vi "final_control_mk11_060325.vi"() -> ()   [LabVIEW 2023]
doc: "Simplified example program for initializing the COM port, determining the data frame of up to 26 Alicats, acquiring the data of the same number of Alicats, displaying the data of the one with the selected unit ID, and writing a setpoint to the same selected unit ID.\n\nThis is a slightly more feature rich version of the Alicat Simplified Driver Example, and contains an example of a method for interfacing with up to 26 Alicats on a single COM port by means of for loops with shift registers to handle sequential commands to each included Alicat. This also contains a method to write a setpoint to the same selected unit.\n\nIf coding for multiple Alicats on a single COM port without the use of for loops with shift registers, ensure that each Alicat command is executed sequentially. Alicat's RS-232/485 does not work if multiple devices are responding simultaneously."
uses:
  <vilib>/Platform/TimedLoop/XDataNode/timing_clust.ctl
  <vilib>/Platform/TimedLoop/XDataNode/nitl_modes.ctl
  <vilib>/Platform/TimedLoop/XDataNode/wakeup.ctl
  <vilib>/DAQmx/write.llb/DAQmx Write (Analog 1D DBL NChan 1Samp).vi
  <vilib>/DAQmx/read.llb/DAQmx Read (Analog DBL 1Chan 1Samp).vi
  <extravilib>/ChannelInstances/Tag-bool/Read With Abort.vi
  <extravilib>/ChannelInstances/Tag-bool/Write With Abort.vi
  <vilib>/Utility/file.llb/Write Delimited Spreadsheet (string).vi
  <extravilib>/ChannelInstances/Tag-bool/Instantiate.vi
  <vilib>/Utility/file.llb/Read Delimited Spreadsheet (DBL).vi
  <extravilib>/ChannelInstances/Tag-bool/EndpointRead.vi
  <vilib>/DAQmx/miscellaneous.llb/DAQmx Fill In Error Info.vi
  <extravilib>/ChannelInstances/Tag-bool/Endpoint.vi
  <vilib>/platform/TimedLoop/XDataNode/XDataNode.xnode
  <vilib>/express/express arith-compare/Formula/XNode/ExpressFormulaBlockNode.xnode
  <vilib>/Platform/TimedLoop/XDataNode/XDNodeRunTimeDep.lvlib
  <extravilib>/ChannelInstances/Tag-bool.lvlib
panel:
  in  "Tab Control":enum32{"Page 1", "Page 2"}(tab)
  in  "COM Port Settings":T1={"Baud Rate"=enum."19200", "VISA Sesssion In"="MassFlowControllers"}
  out "Range Exceeded":bool
  out "Error Present":bool
  out "Error Text":string
  out "Elapsed Time [ms]\n(all units)":dbl caption="Elapsed Time (s)"
  in  "Minimum time between \nreadings [ms] (all units)":u32
  in  "Device ID's \nto Include:":T2={"A"=TRUE, "B"=TRUE, "C"=TRUE, "D"=TRUE, "E"=TRUE, "F"=TRUE, "G"=FALSE, "H"=FALSE, "I"=FALSE, "J"=FALSE, "K"=FALSE, "L"=FALSE, "M"=FALSE, "N"=FALSE, "O"=FALSE, "P"=FALSE, "Q"=FALSE, "R"=FALSE, "S"=FALSE, "T"=FALSE, "U"=FALSE, "V"=FALSE, "W"=FALSE, "X"=FALSE, "Y"=FALSE, "Z"=FALSE}
  out "Active Device":u16(ring) items=["A", "B", "C", "D", "E", "F"]
  out "Meas. Data (for active device)":T3
  in  "Write File":path
  in  "Hold Time\n[min]":dbl=17.0 min=17.0
  out "N":i32
  in  "Read File":path
  in  "End Program":bool
  in  "Start From:":i32=1
  in  "t_read [ms]":dbl=24000.0
  out "T_SCh [C]":dbl format="%0.2f"
  out "iter start":string
  out "Iter_Duration [ms]":string
  out "C_SP [ppm]":string
  out "C_H2 [ppm]":string
  in  "Start Times":path
  in  "API Key":string="V1WFARF28XTM5DW7"
  out "len_SP":i32
  out "Setpoints":dbl[][](array[numeric])=[[4.2, 3.3], [69.0, 4.2]]
  out "Z":dbl[](array[numeric])
  out "ASP":dbl
  out "BSP":dbl
  out "CSP":dbl
  out "DSP":dbl
  out "ESP":dbl
  out "FSP":dbl
  out "N_read":i32
  out "Iter_#":string
  out "V_D":string
  out "V_H":string
  out "all rows":dbl[][](array[numeric])
  out "T_SCh":string
  out "Iteration Duration":i64
  out "read_cnt_true":i32
  out "iter_dur_read [ms]":i64
  out "t_diff":dbl
  out "date":string
  out "time":string
  # "Totalizer Timer"
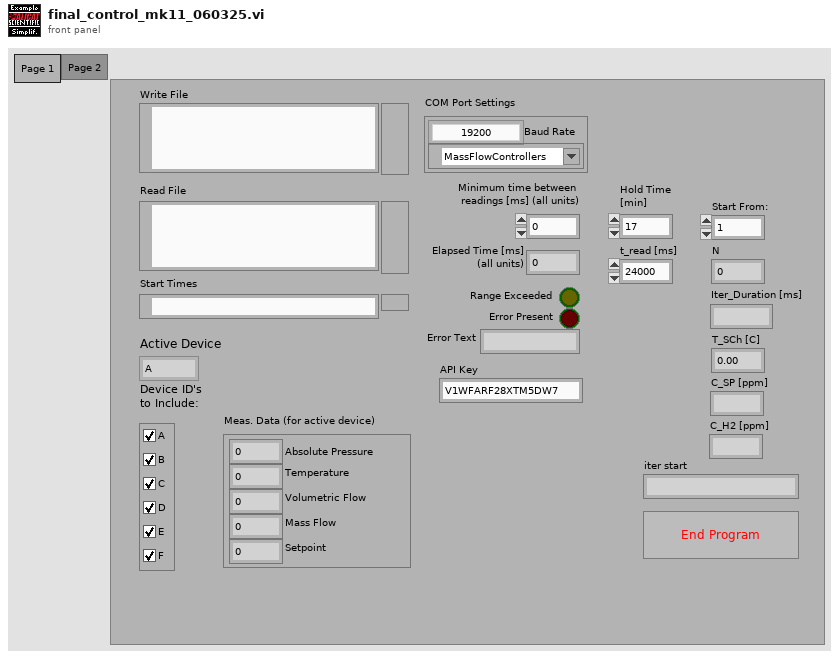
[diagram p1: front panel]
types:
  T1 = cluster{"Baud Rate":enum8{"2400", "9600", "19200", "38400", "57600", "115200", "Unknown"}, "VISA Sesssion In":refnum<visa-resource-name>}
  T2 = cluster{"A":bool, "B":bool, "C":bool, "D":bool, "E":bool, "F":bool, "G":bool, "H":bool, "I":bool, "J":bool, "K":bool, "L":bool, "M":bool, "N":bool, "O":bool, "P":bool, "Q":bool, "R":bool, "S":bool, "T":bool, "U":bool, "V":bool, "W":bool, "X":bool, "Y":bool, "Z":bool}
  T3 = cluster{"Absolute Pressure":dbl, "Gauge/Diff. Pressure":dbl, "Barometric Pressure":dbl, "Temperature":dbl, "Volumetric Flow":dbl, "Mass Flow":dbl, "Setpoint":dbl, "Valve Drive":dbl, "Totalizer":dbl, "[hr]":dbl, "[min]":dbl, "[sec]":dbl, "Totalizer Average Flow":dbl, "Totalizer Peak Flow":dbl, "Gas selected":string}
  T4 = cluster{"Unit ID":string, "Baud Rate":enum8{"2400", "9600", "19200", "38400", "57600", "115200", "Unknown"}, "VISA Sesssion In":refnum<visa-resource-name>}
  T5 = enum16{"Request Ack", "Set Setpoint", "Set Lo Limit", "Set Hi Limit", "Set Prop Band 0-99.9", "Set Integral 0-9.99", "Set Derivative 0-5.0", "Read Int Temp", "Read Ext Temp", "Read Setpoint", "Read Low Limit", "Read High Limit", "Read Prop Band", "Read Integral", "Read Derivative "}
  T6 = typedef "XDNodeRunTimeDep.lvlib/timing_clust.ctl" = cluster{"Expected End [f-1]":u64, "Actual End [f-1]":u64, "Finished Late? [f-1]":bool, "Expected End [i-1]":u64, "Actual End [i-1]":u64, "Finished Late? [i-1]":bool, "Expected Start [i]":u64, "Actual Start [i]":u64, "Expected Start [f]":u64, "Actual Start [f]":u64, "Source Name":string, "Structure Name":string, "Period":i64, "Deadline":i64, "Offset":i64, "Start":i64, "Priority":i32, "Timeout":i32, "Mode":T7, "Wakeup Reason":T8, "Error":errorcluster, "Source Type":string, "Secondary Source Type":string, "Global End Time":u64, "Global Start Time":u64, "Frame Duration":u64, "Iteration Duration":u64, "Assigned CPU":i32, "I/O Scan Engine Mode":u32}
  T7 = typedef "XDNodeRunTimeDep.lvlib/nitl_modes.ctl" = enum32{"No Change", "Process missed periods, maintain original phase", "Discard missed periods, maintain original phase", "Process missed periods, ignore original phase", "Discard missed periods, ignore original phase"}
  T8 = typedef "XDNodeRunTimeDep.lvlib/wakeup.ctl" = enum32{"Normal", "Aborted", "Asynchronous wakeup", "Timing source error", "Timed loop error", "Timeout"}
  T9 = typedef "Tag-bool.lvlib/))Channel.ctl" = refnum<queue>
  T10 = enum8{"2400", "9600", "19200", "38400", "57600", "115200", "Unknown"}
  T11 = cluster{"Absolute Pressure":bool, "Gauge/Diff. Pressure":bool, "Barometric Pressure":bool, "Temperature":bool, "Volumetric":bool, "Mass":bool, "Setpoint":bool, "Valve Drive":bool, "Totalizer":bool, "Totalizer Timer":bool, "Totalizer Average Flow":bool, "Totalizer Peak Flow":bool, "Gas Selected":bool, "Tot. Timer Format":u16}
  T12 = cluster{"Controller Full Scale":dbl, "Controller Select":u16, "Control Range":enum16{"Normal", "Inverted", "Bidirectional", "Unknown"}}
  T13 = cluster{"Controller Full Scale":dbl, "Controller Select":u16, "Control Range":enum16{"Normal", "Inverted", "Bidirectional", "Unknown"}}[]
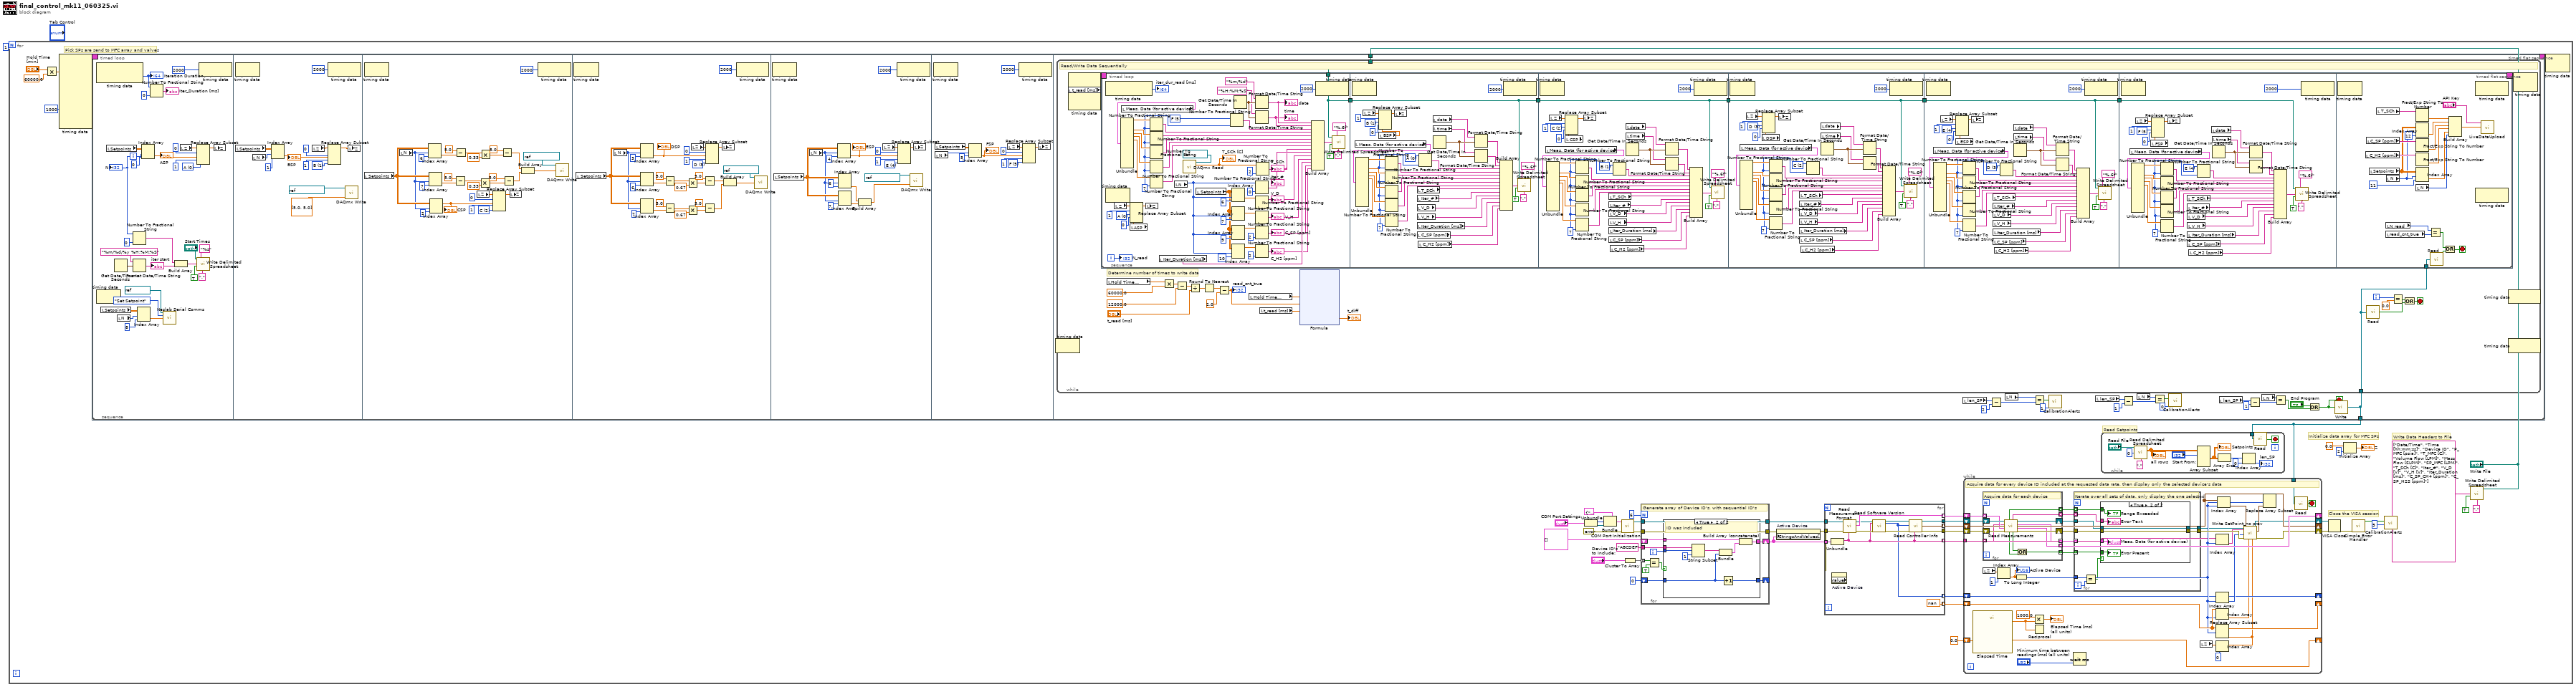
[diagram p0: block diagram]
diagram:
  n1 = for {
    N: 1 -> [_]
    # "Pick SPs are send to MFC array and valves"
    # "Write Data Headers to File"
    # "Read Setpoints"
    # "Initialize data array for MFC SPs"
    # "Close the VISA session"
    n2 = Multiply(x="Hold Time\n[min]", y=60000.0) -> (x*y=w5:dbl)
    n3 = node-c288(w5, i64 1000 ("Offset")) -> (w46:T6)  [unwired: 8 in]
    n4 = timed-loop "Write Data" {
      timing: w46 -> [_]
      timing-out: [_] -> w45
      tunnel: [w59] -> w12
      tunnel: "Write File" -> [w58]
      i -> [w73]
      stop <- w227 stop-if-true
      n5 = timed-sequence {
        timing: _ -> [_]
        timing-out: _ -> [_]
        tunnel: [w61] -> w59
        tunnel: w58 -> [w60]
        n6 = timed-flat-sequence {
          tunnel: [w222] -> w61
          tunnel: w60 -> [w223]
          frame #0 {
            w83 = u16 0 items=["A", "B", "C", "D", "E", "F"]
            n7 = node-c288() -> (w77:i64)  [unwired: 1 in, 1 out]
            "Iteration Duration" <- w77
            n8 = local read "Setpoints"() -> (w67:dbl[][])
            n9 = local read "Setpoints"() -> (w90:dbl[][])
            n10 = Get Date/Time In Seconds() -> (seconds since 1Jan1904=w78:timestamp)
            n11 = local read "N"() -> (w66:i32)
            n12 = Number To Fractional String(number=w73, precision (6)=i16 0) -> (F-format string=w71:string)  [unwired: 2 in]
            n13 = Format Date/Time String(time format string (%c)="%m/%d/%y %H:%M:%S", seconds (now)=w78) -> (date/time string=w70:string)  [unwired: 1 in]
            "iter start" <- w70
            n14 = Index Array(array=w67, index (row)=w66, index (col)=8 ("disabled index (col)")) -> (element=w64:dbl)
            n15 = Index Array(array=w90, index (row)=w73, index (col)=0 ("index (row)")) -> (element=w88:dbl)
            "ASP" <- w88
            n16 = Number To Fractional String(number=w77, precision (6)=i16 0) -> (F-format string=→"Iter_Duration [ms]":string)  [unwired: 2 in]
            n17 = call "Neslab Serial Comms.vi"("VISA resource name"=refnum<visa-resource-name> "COM1", "Command"=T5."Set Setpoint", "Set Value"=w64) -> ()  [unwired: 6 in, 7 out]
            n18 = Build Array(w71, w70) -> (w69:string[])
            n19 = local read "Z"() -> (w86:dbl[])
            n20 = Replace Array Subset(array=w86, new element #1=w88, index #1=0 ("index"), new element #2=w83, index #2=1 ("index")) -> (w87:dbl[])
            n21 = call-poly <vilib>:"Write Delimited Spreadsheet.vi"("file path (dialog if empty)"="Start Times", "format (%s)"="%s" ("format (%.3f)"), "1D data"=w69, "append to file? (new file:F)"=TRUE, "delimiter (\\t)"="," ("delimiter (\\t)")) -> ()  [unwired: 9 in, 2 out]
            n22 = node-c288(i64 2000 ("Start")) -> ()  [unwired: 1 out]
            n23 = local write "Z"(w87) -> ()
            "N" <- w73
          }
          frame #1 {
            w98 = u16 1 items=["A", "B", "C", "D", "E", "F"]
            n24 = node-c288() -> ()  [unwired: 1 in, 1 out]
            n25 = local read "Setpoints"() -> (w106:dbl[][])
            n26 = local read "N"() -> (w99:i32)
            n27 = Index Array(array=w106, index (row)=w99, index (col)=1 ("index (row)")) -> (element=w103:dbl)
            "BSP" <- w103
            n28 = local read "Z"() -> (w101:dbl[])
            n29 = Replace Array Subset(array=w101, new element #1=w103, index #1=0 ("index"), new element #2=w98, index #2=1 ("index")) -> (w102:dbl[])
            n30 = node-c288(i64 2000 ("Start")) -> ()  [unwired: 1 out]
            n31 = call-poly <vilib>:"DAQmx Write.vi"("task/channels in"=refnum<k21> "Valve_cont", "data"=dbl[] [5.0, 5.0]) -> ()  [unwired: 11 in, 3 out]
            n32 = local write "Z"(w102) -> ()
          }
          frame #2 {
            w113 = u16 2 items=["A", "B", "C", "D", "E", "F"]
            n33 = node-c288() -> ()  [unwired: 1 in, 1 out]
            n34 = local read "Setpoints"() -> (w125:dbl[][])
            n35 = local read "N"() -> (w124:i32)
            n36 = Index Array(array=w125, index (row)=w124, index (col)=6 ("disabled index (col)")) -> (element=w115:dbl)
            n37 = Index Array(array=w125, index (row)=w124, index (col)=7 ("disabled index (col)")) -> (element=w123:dbl)
            n38 = Index Array(array=w125, index (row)=w124, index (col)=2 ("index (row)")) -> (element=w137:dbl)
            "CSP" <- w137
            n39 = Subtract(x=5.0, y=w123) -> (x-y=w132:dbl)
            n40 = Subtract(x=5.0, y=w115) -> (x-y=w119:dbl)
            n41 = local read "Z"() -> (w135:dbl[])
            n42 = Multiply(x=w132, y=0.33) -> (x*y=w130:dbl)
            n43 = Multiply(x=w119, y=0.33) -> (x*y=w117:dbl)
            n44 = Replace Array Subset(array=w135, new element #1=w137, index #1=0 ("index"), new element #2=w113, index #2=1 ("index")) -> (w136:dbl[])
            n45 = Subtract(x=5.0, y=w117) -> (x-y=w114:dbl)
            n46 = Subtract(x=5.0, y=w130) -> (x-y=w127:dbl)
            n47 = local write "Z"(w136) -> ()
            n48 = Build Array(w114, w127) -> (w126:dbl[])
            n49 = node-c288(i64 2000 ("Start")) -> ()  [unwired: 1 out]
            n50 = call-poly <vilib>:"DAQmx Write.vi"("task/channels in"=refnum<k21> "Valve_cont", "data"=w126) -> ()  [unwired: 11 in, 3 out]
          }
          frame #3 {
            w164 = u16 3 items=["A", "B", "C", "D", "E", "F"]
            n51 = node-c288() -> ()  [unwired: 1 in, 1 out]
            n52 = local read "Setpoints"() -> (w153:dbl[][])
            n53 = local read "N"() -> (w152:i32)
            n54 = Index Array(array=w153, index (row)=w152, index (col)=7 ("disabled index (col)")) -> (element=w145:dbl)
            n55 = Index Array(array=w153, index (row)=w152, index (col)=3 ("index (row)")) -> (element=w168:dbl)
            "DSP" <- w168
            n56 = Index Array(array=w153, index (row)=w152, index (col)=6 ("disabled index (col)")) -> (element=w151:dbl)
            n57 = Subtract(x=5.0, y=w151) -> (x-y=w161:dbl)
            n58 = Subtract(x=5.0, y=w145) -> (x-y=w149:dbl)
            n59 = Multiply(x=w161, y=0.67) -> (x*y=w159:dbl)
            n60 = Multiply(x=w149, y=0.67) -> (x*y=w147:dbl)
            n61 = local read "Z"() -> (w166:dbl[])
            n62 = Subtract(x=5.0, y=w159) -> (x-y=w155:dbl)
            n63 = Subtract(x=5.0, y=w147) -> (x-y=w144:dbl)
            n64 = Replace Array Subset(array=w166, new element #1=w168, index #1=0 ("index"), new element #2=w164, index #2=1 ("index")) -> (w167:dbl[])
            n65 = local write "Z"(w167) -> ()
            n66 = Build Array(w155, w144) -> (w154:dbl[])
            n67 = node-c288(i64 2000 ("Start")) -> ()  [unwired: 1 out]
            n68 = call-poly <vilib>:"DAQmx Write.vi"("task/channels in"=refnum<k21> "Valve_cont", "data"=w154) -> ()  [unwired: 11 in, 3 out]
          }
          frame #4 {
            w185 = u16 4 items=["A", "B", "C", "D", "E", "F"]
            n69 = node-c288() -> ()  [unwired: 1 in, 1 out]
            n70 = local read "Setpoints"() -> (w180:dbl[][])
            n71 = local read "N"() -> (w179:i32)
            n72 = Index Array(array=w180, index (row)=w179, index (col)=4 ("index (row)")) -> (element=w189:dbl)
            "ESP" <- w189
            n73 = Index Array(array=w180, index (row)=w179, index (col)=6 ("disabled index (col)")) -> (element=w182:dbl)
            n74 = Index Array(array=w180, index (row)=w179, index (col)=7 ("disabled index (col)")) -> (element=w181:dbl)
            n75 = Build Array(w182, w181) -> (w178:dbl[])
            n76 = local read "Z"() -> (w187:dbl[])
            n77 = node-c288(i64 2000 ("Start")) -> ()  [unwired: 1 out]
            n78 = Replace Array Subset(array=w187, new element #1=w189, index #1=0 ("index"), new element #2=w185, index #2=1 ("index")) -> (w188:dbl[])
            n79 = call-poly <vilib>:"DAQmx Write.vi"("task/channels in"=refnum<k21> "Valve_cont", "data"=w178) -> ()  [unwired: 11 in, 3 out]
            n80 = local write "Z"(w188) -> ()
          }
          frame #5 {
            w199 = u16 5 items=["A", "B", "C", "D", "E", "F"]
            n81 = node-c288() -> ()  [unwired: 1 in, 1 out]
            n82 = local read "Setpoints"() -> (w202:dbl[][])
            n83 = local read "N"() -> (w197:i32)
            n84 = Index Array(array=w202, index (row)=w197, index (col)=5 ("index (row)")) -> (element=w198:dbl)
            "FSP" <- w198
            n85 = local read "Z"() -> (w201:dbl[])
            n86 = node-c288(i64 2000 ("Start")) -> ()  [unwired: 1 out]
            n87 = Replace Array Subset(array=w201, new element #1=w198, index #1=0 ("index"), new element #2=w199, index #2=1 ("index")) -> (w200:dbl[])
            n88 = local write "Z"(w200) -> ()
          }
          frame #6 {
            n89 = node-c288() -> ()  [unwired: 1 in, 1 out]
            n90 = local read "len_SP"() -> (w213:i32)
            n91 = Subtract(x=w213, y=2) -> (x-y=w215:i32)
            n92 = local read "N"() -> (w214:i32)
            n93 = Equal?(x=w214, y=w215) -> (x = y?=w211:bool)
            n94 = call "CalibrationAlerts.vi"("Alert Type (0)"=1, "Trigger"=w211) -> ()  [unwired: 10 in]
            n95 = local read "len_SP"() -> (w218:i32)
            n96 = Subtract(x=w218, y=1) -> (x-y=w217:i32)
            n97 = local read "N"() -> (w221:i32)
            n98 = Equal?(x=w221, y=w217) -> (x = y?=w210:bool)
            n99 = call "CalibrationAlerts.vi"("Alert Type (0)"=0, "Trigger"=w210) -> ()  [unwired: 10 in]
            n100 = local read "len_SP"() -> (w226:i32)
            n101 = Subtract(x=w226, y=1) -> (x-y=w229:i32)
            n102 = local read "N"() -> (w225:i32)
            n103 = Equal?(x=w225, y=w229) -> (x = y?=w228:bool)
            n104 = Or(x="End Program", y=w228) -> (x .or. y?=w227:bool)
            n105 = call <extravilib>:"Write.vi"("element"=w227) -> ("channel"=w222:T9)  [unwired: 1 out]
            n106 = while {
              tunnel: w223 -> [w251]
              tunnel: w222 -> [w241]
              i -> [w240]
              stop <- w247 stop-if-true
              # "Determine number of times to write data"
              # "Read/Write Data Sequentially"
              n107 = local read "t_read [ms]"() -> (w231:dbl)
              n108 = node-c288(w231) -> (w253:T6)  [unwired: 3 in]
              n109 = timed-loop {
                timing: w253 -> [_]
                timing-out: [_] -> w252
                tunnel: w251 -> [w266]
                tunnel: w241 -> [w267]
                i -> [w330]
                stop <- w564 stop-if-true
                n110 = timed-sequence {
                  timing: _ -> [_]
                  timing-out: _ -> [_]
                  tunnel: w267 -> [w269]
                  tunnel: w266 -> [w268]
                  n111 = timed-flat-sequence {
                    tunnel: [w296] -> w274
                    tunnel: w268 -> [w296]
                    tunnel: w274 -> [w361]
                    tunnel: [w361] -> w273
                    tunnel: w273 -> [w396]
                    tunnel: [w396] -> w272
                    tunnel: w272 -> [w434]
                    tunnel: [w434] -> w271
                    tunnel: w271 -> [w466]
                    tunnel: [w466] -> w270
                    tunnel: w270 -> [w519]
                    tunnel: w269 -> [w563]
                    frame #0 {
                      w311 = u16 5 items=["A", "B", "C", "D", "E", "F"]
                      w314 = u16 0 items=["A", "B", "C", "D", "E", "F"]
                      w307 = i16 7 ("precision (6)")
                      n112 = node-c288() -> (→"iter_dur_read [ms]":i64)  [unwired: 1 in]
                      n113 = local read "Z"() -> (w300:dbl[])
                      n114 = local read "Meas. Data (for active device)"() -> (w297:T3)
                      n115 = Unbundle(w297) -> ("Absolute Pressure"=w320:dbl, "Temperature"=w310:dbl, "Volumetric Flow"=w316:dbl, "Mass Flow"=w309:dbl, "Setpoint"=w308:dbl)  [unwired: 10 out]
                      n116 = local read "ASP"() -> (w298:dbl)
                      n117 = Replace Array Subset(array=w300, new element #1=w314, index #1=1 ("index"), new element #2=w298, index #2=0 ("index")) -> (w299:dbl[])
                      n118 = local write "Z"(w299) -> ()
                      n119 = Number To Fractional String(number=w320, precision (6)=w307) -> (F-format string=w305:string)  [unwired: 2 in]
                      n120 = Number To Fractional String(number=w310, precision (6)=w307) -> (F-format string=w303:string)  [unwired: 2 in]
                      n121 = Number To Fractional String(number=w316, precision (6)=w307) -> (F-format string=w304:string)  [unwired: 2 in]
                      n122 = Number To Fractional String(number=w309, precision (6)=w307) -> (F-format string=w302:string)  [unwired: 2 in]
                      n123 = Number To Fractional String(number=w308, precision (6)=w307) -> (F-format string=w301:string)  [unwired: 2 in]
                      n124 = local read "Iter_Duration [ms]"() -> (w295:string)
                      n125 = local read "N"() -> (w277:i32)
                      n126 = call-poly <vilib>:"DAQmx Read.vi"("task/channels in"=refnum<k21> "Temp") -> ("data"=w323:dbl)  [unwired: 12 in, 2 out]
                      "T_SCh [C]" <- w323
                      n127 = local read "Setpoints"() -> (w276:dbl[][])
                      n128 = Number To Fractional String(number=w311, precision (6)=w307) -> (F-format string=w306:string)  [unwired: 2 in]
                      n129 = Index Array(array=w276, index (row)=w277, index (col)=6 ("disabled index (col)")) -> (element=w327:dbl)
                      n130 = Index Array(array=w276, index (row)=w277, index (col)=7 ("disabled index (col)")) -> (element=w326:dbl)
                      n131 = Index Array(array=w276, index (row)=w277, index (col)=9 ("disabled index (col)")) -> (element=w283:dbl)
                      n132 = Index Array(array=w276, index (row)=w277, index (col)=10 ("disabled index (col)")) -> (element=w279:dbl)
                      n133 = Get Date/Time In Seconds() -> (seconds since 1Jan1904=w289:timestamp)
                      n134 = Format Date/Time String(time format string (%c)="%m/%d", seconds (now)=w289) -> (date/time string=w291:string)  [unwired: 1 in]
                      "date" <- w291
                      n135 = Format Date/Time String(time format string (%c)="%H:%M:%S", seconds (now)=w289) -> (date/time string=w290:string)  [unwired: 1 in]
                      "time" <- w290
                      n136 = Number To Fractional String(number=w277, precision (6)=i16 0) -> (F-format string=w292:string)  [unwired: 2 in]
                      "Iter_#" <- w292
                      n137 = Number To Fractional String(number=w327) -> (F-format string=w293:string)  [unwired: 3 in]
                      "V_D" <- w293
                      n138 = Number To Fractional String(number=w326) -> (F-format string=w294:string)  [unwired: 3 in]
                      "V_H" <- w294
                      n139 = Number To Fractional String(number=w283, precision (6)=i16 2) -> (F-format string=w281:string)  [unwired: 2 in]
                      "C_SP [ppm]" <- w281
                      n140 = Number To Fractional String(number=w279, precision (6)=i16 2) -> (F-format string=w275:string)  [unwired: 2 in]
                      "C_H2 [ppm]" <- w275
                      n141 = Number To Fractional String(number=w323, precision (6)=i16 2) -> (F-format string=w286:string)  [unwired: 2 in]
                      "T_SCh" <- w286
                      n142 = Build Array(w291, w290, w306, w305, w303, w304, w302, w301, w286, w292, w293, w294, w295, w281, w275) -> (w317:string[])
                      n143 = node-c288(i64 2000 ("Start")) -> ()  [unwired: 1 out]
                      n144 = call-poly <vilib>:"Write Delimited Spreadsheet.vi"("file path (dialog if empty)"=w296, "format (%s)"="%.6f" ("format (%.3f)"), "1D data"=w317, "append to file? (new file:F)"=TRUE, "delimiter (\\t)"="," ("delimiter (\\t)")) -> ()  [unwired: 9 in, 2 out]
                      "N_read" <- w330
                    }
                    frame #1 {
                      w358 = u16 0 items=["A", "B", "C", "D", "E", "F"]
                      w367 = u16 1 items=["A", "B", "C", "D", "E", "F"]
                      w354 = i16 7 ("precision (6)")
                      n145 = node-c288() -> ()  [unwired: 1 in, 1 out]
                      n146 = local read "Meas. Data (for active device)"() -> (w365:T3)
                      n147 = Unbundle(w365) -> ("Absolute Pressure"=w373:dbl, "Temperature"=w357:dbl, "Volumetric Flow"=w369:dbl, "Mass Flow"=w356:dbl, "Setpoint"=w355:dbl)  [unwired: 10 out]
                      n148 = local read "Z"() -> (w364:dbl[])
                      n149 = local read "BSP"() -> (w359:dbl)
                      n150 = Replace Array Subset(array=w364, new element #1=w367, index #1=1 ("index"), new element #2=w359, index #2=0 ("index")) -> (w363:dbl[])
                      n151 = Number To Fractional String(number=w373, precision (6)=w354) -> (F-format string=w352:string)  [unwired: 2 in]
                      n152 = Number To Fractional String(number=w357, precision (6)=w354) -> (F-format string=w350:string)  [unwired: 2 in]
                      n153 = Number To Fractional String(number=w369, precision (6)=w354) -> (F-format string=w351:string)  [unwired: 2 in]
                      n154 = Number To Fractional String(number=w356, precision (6)=w354) -> (F-format string=w349:string)  [unwired: 2 in]
                      n155 = Number To Fractional String(number=w355, precision (6)=w354) -> (F-format string=w348:string)  [unwired: 2 in]
                      n156 = local write "Z"(w363) -> ()
                      n157 = local read "T_SCh"() -> (w347:string)
                      n158 = local read "Iter_#"() -> (w346:string)
                      n159 = local read "V_D"() -> (w345:string)
                      n160 = local read "V_H"() -> (w344:string)
                      n161 = local read "Iter_Duration [ms]"() -> (w343:string)
                      n162 = local read "C_SP [ppm]"() -> (w337:string)
                      n163 = local read "C_H2 [ppm]"() -> (w336:string)
                      n164 = Number To Fractional String(number=w358, precision (6)=w354) -> (F-format string=w353:string)  [unwired: 2 in]
                      n165 = local read "date"() -> (w338:string)
                      n166 = local read "time"() -> (w339:string)
                      n167 = Get Date/Time In Seconds() -> (seconds since 1Jan1904=w340:timestamp)
                      n168 = Format Date/Time String(time format string (%c)=w338, seconds (now)=w340) -> (date/time string=w342:string)  [unwired: 1 in]
                      n169 = Format Date/Time String(time format string (%c)=w339, seconds (now)=w340) -> (date/time string=w341:string)  [unwired: 1 in]
                      n170 = Build Array(w342, w341, w353, w352, w350, w351, w349, w348, w347, w346, w345, w344, w343, w337, w336) -> (w370:string[])
                      n171 = node-c288(i64 2000 ("Start")) -> ()  [unwired: 1 out]
                      n172 = call-poly <vilib>:"Write Delimited Spreadsheet.vi"("file path (dialog if empty)"=w361, "format (%s)"="%.6f" ("format (%.3f)"), "1D data"=w370, "append to file? (new file:F)"=TRUE, "delimiter (\\t)"="," ("delimiter (\\t)")) -> ()  [unwired: 9 in, 2 out]
                    }
                    frame #2 {
                      w402 = u16 1 items=["A", "B", "C", "D", "E", "F"]
                      w401 = i16 7 ("precision (6)")
                      w414 = u16 2 items=["A", "B", "C", "D", "E", "F"]
                      n173 = node-c288() -> ()  [unwired: 1 in, 1 out]
                      n174 = local read "Meas. Data (for active device)"() -> (w403:T3)
                      n175 = Unbundle(w403) -> ("Absolute Pressure"=w408:dbl, "Temperature"=w406:dbl, "Volumetric Flow"=w407:dbl, "Mass Flow"=w405:dbl, "Setpoint"=w404:dbl)  [unwired: 10 out]
                      n176 = local read "Z"() -> (w413:dbl[])
                      n177 = local read "CSP"() -> (w409:dbl)
                      n178 = Replace Array Subset(array=w413, new element #1=w414, index #1=1 ("index"), new element #2=w409, index #2=0 ("index")) -> (w412:dbl[])
                      n179 = Number To Fractional String(number=w408, precision (6)=w401) -> (F-format string=w389:string)  [unwired: 2 in]
                      n180 = Number To Fractional String(number=w406, precision (6)=w401) -> (F-format string=w388:string)  [unwired: 2 in]
                      n181 = Number To Fractional String(number=w407, precision (6)=w401) -> (F-format string=w387:string)  [unwired: 2 in]
                      n182 = Number To Fractional String(number=w405, precision (6)=w401) -> (F-format string=w386:string)  [unwired: 2 in]
                      n183 = Number To Fractional String(number=w404, precision (6)=w401) -> (F-format string=w385:string)  [unwired: 2 in]
                      n184 = local write "Z"(w412) -> ()
                      n185 = local read "T_SCh"() -> (w395:string)
                      n186 = local read "Iter_#"() -> (w394:string)
                      n187 = local read "V_D"() -> (w393:string)
                      n188 = local read "V_H"() -> (w392:string)
                      n189 = local read "Iter_Duration [ms]"() -> (w391:string)
                      n190 = local read "C_SP [ppm]"() -> (w379:string)
                      n191 = local read "C_H2 [ppm]"() -> (w378:string)
                      n192 = Number To Fractional String(number=w402, precision (6)=w401) -> (F-format string=w390:string)  [unwired: 2 in]
                      n193 = local read "date"() -> (w380:string)
                      n194 = local read "time"() -> (w381:string)
                      n195 = Get Date/Time In Seconds() -> (seconds since 1Jan1904=w382:timestamp)
                      n196 = Format Date/Time String(time format string (%c)=w380, seconds (now)=w382) -> (date/time string=w384:string)  [unwired: 1 in]
                      n197 = Format Date/Time String(time format string (%c)=w381, seconds (now)=w382) -> (date/time string=w383:string)  [unwired: 1 in]
                      n198 = Build Array(w384, w383, w390, w389, w388, w387, w386, w385, w395, w394, w393, w392, w391, w379, w378) -> (w397:string[])
                      n199 = node-c288(i64 2000 ("Start")) -> ()  [unwired: 1 out]
                      n200 = call-poly <vilib>:"Write Delimited Spreadsheet.vi"("file path (dialog if empty)"=w396, "format (%s)"="%.6f" ("format (%.3f)"), "1D data"=w397, "append to file? (new file:F)"=TRUE, "delimiter (\\t)"="," ("delimiter (\\t)")) -> ()  [unwired: 9 in, 2 out]
                    }
                    frame #3 {
                      w428 = u16 3 items=["A", "B", "C", "D", "E", "F"]
                      w451 = u16 2 items=["A", "B", "C", "D", "E", "F"]
                      w450 = i16 7 ("precision (6)")
                      n201 = node-c288() -> ()  [unwired: 1 in, 1 out]
                      n202 = local read "Meas. Data (for active device)"() -> (w433:T3)
                      n203 = Unbundle(w433) -> ("Absolute Pressure"=w456:dbl, "Temperature"=w454:dbl, "Volumetric Flow"=w455:dbl, "Mass Flow"=w453:dbl, "Setpoint"=w452:dbl)  [unwired: 10 out]
                      n204 = local read "Z"() -> (w431:dbl[])
                      n205 = local read "DSP"() -> (w432:dbl)
                      n206 = Replace Array Subset(array=w431, new element #1=w428, index #1=1 ("index"), new element #2=w432, index #2=0 ("index")) -> (w430:dbl[])
                      n207 = Number To Fractional String(number=w456, precision (6)=w450) -> (F-format string=w444:string)  [unwired: 2 in]
                      n208 = Number To Fractional String(number=w454, precision (6)=w450) -> (F-format string=w443:string)  [unwired: 2 in]
                      n209 = Number To Fractional String(number=w455, precision (6)=w450) -> (F-format string=w442:string)  [unwired: 2 in]
                      n210 = Number To Fractional String(number=w453, precision (6)=w450) -> (F-format string=w441:string)  [unwired: 2 in]
                      n211 = Number To Fractional String(number=w452, precision (6)=w450) -> (F-format string=w440:string)  [unwired: 2 in]
                      n212 = local write "Z"(w430) -> ()
                      n213 = local read "T_SCh"() -> (w435:string)
                      n214 = local read "Iter_#"() -> (w436:string)
                      n215 = local read "V_D"() -> (w437:string)
                      n216 = local read "V_H"() -> (w438:string)
                      n217 = local read "Iter_Duration [ms]"() -> (w439:string)
                      n218 = local read "C_SP [ppm]"() -> (w421:string)
                      n219 = local read "C_H2 [ppm]"() -> (w420:string)
                      n220 = Number To Fractional String(number=w451, precision (6)=w450) -> (F-format string=w445:string)  [unwired: 2 in]
                      n221 = local read "date"() -> (w422:string)
                      n222 = local read "time"() -> (w423:string)
                      n223 = Get Date/Time In Seconds() -> (seconds since 1Jan1904=w424:timestamp)
                      n224 = Format Date/Time String(time format string (%c)=w422, seconds (now)=w424) -> (date/time string=w426:string)  [unwired: 1 in]
                      n225 = Format Date/Time String(time format string (%c)=w423, seconds (now)=w424) -> (date/time string=w425:string)  [unwired: 1 in]
                      n226 = Build Array(w426, w425, w445, w444, w443, w442, w441, w440, w435, w436, w437, w438, w439, w421, w420) -> (w446:string[])
                      n227 = node-c288(i64 2000 ("Start")) -> ()  [unwired: 1 out]
                      n228 = call-poly <vilib>:"Write Delimited Spreadsheet.vi"("file path (dialog if empty)"=w434, "format (%s)"="%.6f" ("format (%.3f)"), "1D data"=w446, "append to file? (new file:F)"=TRUE, "delimiter (\\t)"="," ("delimiter (\\t)")) -> ()  [unwired: 9 in, 2 out]
                    }
                    frame #4 {
                      w474 = u16 4 items=["A", "B", "C", "D", "E", "F"]
                      w493 = u16 3 items=["A", "B", "C", "D", "E", "F"]
                      w492 = i16 7 ("precision (6)")
                      n229 = node-c288() -> ()  [unwired: 1 in, 1 out]
                      n230 = local read "Meas. Data (for active device)"() -> (w476:T3)
                      n231 = Unbundle(w476) -> ("Absolute Pressure"=w498:dbl, "Temperature"=w496:dbl, "Volumetric Flow"=w497:dbl, "Mass Flow"=w495:dbl, "Setpoint"=w494:dbl)  [unwired: 10 out]
                      n232 = local read "Z"() -> (w471:dbl[])
                      n233 = local read "ESP"() -> (w472:dbl)
                      n234 = Replace Array Subset(array=w471, new element #1=w474, index #1=1 ("index"), new element #2=w472, index #2=0 ("index")) -> (w470:dbl[])
                      n235 = Number To Fractional String(number=w498, precision (6)=w492) -> (F-format string=w486:string)  [unwired: 2 in]
                      n236 = Number To Fractional String(number=w496, precision (6)=w492) -> (F-format string=w485:string)  [unwired: 2 in]
                      n237 = Number To Fractional String(number=w497, precision (6)=w492) -> (F-format string=w484:string)  [unwired: 2 in]
                      n238 = Number To Fractional String(number=w495, precision (6)=w492) -> (F-format string=w483:string)  [unwired: 2 in]
                      n239 = Number To Fractional String(number=w494, precision (6)=w492) -> (F-format string=w482:string)  [unwired: 2 in]
                      n240 = local write "Z"(w470) -> ()
                      n241 = local read "T_SCh"() -> (w481:string)
                      n242 = local read "Iter_#"() -> (w477:string)
                      n243 = local read "V_D"() -> (w478:string)
                      n244 = local read "V_H"() -> (w479:string)
                      n245 = local read "Iter_Duration [ms]"() -> (w480:string)
                      n246 = local read "C_SP [ppm]"() -> (w463:string)
                      n247 = local read "C_H2 [ppm]"() -> (w462:string)
                      n248 = Number To Fractional String(number=w493, precision (6)=w492) -> (F-format string=w487:string)  [unwired: 2 in]
                      n249 = local read "date"() -> (w464:string)
                      n250 = local read "time"() -> (w465:string)
                      n251 = Get Date/Time In Seconds() -> (seconds since 1Jan1904=w467:timestamp)
                      n252 = Format Date/Time String(time format string (%c)=w464, seconds (now)=w467) -> (date/time string=w469:string)  [unwired: 1 in]
                      n253 = Format Date/Time String(time format string (%c)=w465, seconds (now)=w467) -> (date/time string=w468:string)  [unwired: 1 in]
                      n254 = Build Array(w469, w468, w487, w486, w485, w484, w483, w482, w481, w477, w478, w479, w480, w463, w462) -> (w488:string[])
                      n255 = node-c288(i64 2000 ("Start")) -> ()  [unwired: 1 out]
                      n256 = call-poly <vilib>:"Write Delimited Spreadsheet.vi"("file path (dialog if empty)"=w466, "format (%s)"="%.6f" ("format (%.3f)"), "1D data"=w488, "append to file? (new file:F)"=TRUE, "delimiter (\\t)"="," ("delimiter (\\t)")) -> ()  [unwired: 9 in, 2 out]
                    }
                    frame #5 {
                      w517 = u16 5 items=["A", "B", "C", "D", "E", "F"]
                      w536 = u16 4 items=["A", "B", "C", "D", "E", "F"]
                      w535 = i16 7 ("precision (6)")
                      n257 = node-c288() -> ()  [unwired: 1 in, 1 out]
                      n258 = local read "Meas. Data (for active device)"() -> (w520:T3)
                      n259 = Unbundle(w520) -> ("Absolute Pressure"=w541:dbl, "Temperature"=w539:dbl, "Volumetric Flow"=w540:dbl, "Mass Flow"=w538:dbl, "Setpoint"=w537:dbl)  [unwired: 10 out]
                      n260 = local read "Z"() -> (w513:dbl[])
                      n261 = local read "FSP"() -> (w515:dbl)
                      n262 = Replace Array Subset(array=w513, new element #1=w517, index #1=1 ("index"), new element #2=w515, index #2=0 ("index")) -> (w514:dbl[])
                      n263 = Number To Fractional String(number=w541, precision (6)=w535) -> (F-format string=w529:string)  [unwired: 2 in]
                      n264 = Number To Fractional String(number=w539, precision (6)=w535) -> (F-format string=w528:string)  [unwired: 2 in]
                      n265 = Number To Fractional String(number=w540, precision (6)=w535) -> (F-format string=w527:string)  [unwired: 2 in]
                      n266 = Number To Fractional String(number=w538, precision (6)=w535) -> (F-format string=w526:string)  [unwired: 2 in]
                      n267 = Number To Fractional String(number=w537, precision (6)=w535) -> (F-format string=w525:string)  [unwired: 2 in]
                      n268 = local write "Z"(w514) -> ()
                      n269 = local read "T_SCh"() -> (w504:string)
                      n270 = local read "Iter_#"() -> (w521:string)
                      n271 = local read "V_D"() -> (w522:string)
                      n272 = local read "V_H"() -> (w523:string)
                      n273 = local read "Iter_Duration [ms]"() -> (w524:string)
                      n274 = local read "C_SP [ppm]"() -> (w507:string)
                      n275 = local read "C_H2 [ppm]"() -> (w506:string)
                      n276 = Number To Fractional String(number=w536, precision (6)=w535) -> (F-format string=w530:string)  [unwired: 2 in]
                      n277 = local read "date"() -> (w508:string)
                      n278 = local read "time"() -> (w509:string)
                      n279 = Get Date/Time In Seconds() -> (seconds since 1Jan1904=w510:timestamp)
                      n280 = Format Date/Time String(time format string (%c)=w508, seconds (now)=w510) -> (date/time string=w512:string)  [unwired: 1 in]
                      n281 = Format Date/Time String(time format string (%c)=w509, seconds (now)=w510) -> (date/time string=w511:string)  [unwired: 1 in]
                      n282 = Build Array(w512, w511, w530, w529, w528, w527, w526, w525, w504, w521, w522, w523, w524, w507, w506) -> (w531:string[])
                      n283 = call-poly <vilib>:"Write Delimited Spreadsheet.vi"("file path (dialog if empty)"=w519, "format (%s)"="%.6f" ("format (%.3f)"), "1D data"=w531, "append to file? (new file:F)"=TRUE, "delimiter (\\t)"="," ("delimiter (\\t)")) -> ()  [unwired: 9 in, 2 out]
                      n284 = node-c288(i64 2000 ("Start")) -> ()  [unwired: 1 out]
                    }
                    frame #6 {
                      n285 = node-c288() -> ()  [unwired: 1 in, 1 out]
                      n286 = local read "C_H2 [ppm]"() -> (w556:string)
                      n287 = local read "C_SP [ppm]"() -> (w557:string)
                      n288 = local read "Setpoints"() -> (w554:dbl[][])
                      n289 = local read "T_SCh"() -> (w559:string)
                      n290 = local read "N_read"() -> (w561:i32)
                      n291 = local read "read_cnt_true"() -> (w562:i32)
                      n292 = local read "N"() -> (w553:i32)
                      n293 = Fract/Exp String To Number(string=w559) -> (number=w558:dbl)  [unwired: 3 in, 1 out]
                      n294 = Index Array(array=w554, index (row)=w553, index (col)=12 ("disabled index (col)")) -> (element=w551:dbl)
                      n295 = Fract/Exp String To Number(string=w557) -> (number=w550:dbl)  [unwired: 3 in, 1 out]
                      n296 = Fract/Exp String To Number(string=w556) -> (number=w549:dbl)  [unwired: 3 in, 1 out]
                      n297 = Index Array(array=w554, index (row)=w553, index (col)=11 ("disabled index (col)")) -> (element=w548:dbl)
                      n298 = local read "N"() -> (w547:i32)
                      n299 = Equal?(x=w561, y=w562) -> (x = y?=w566:bool)
                      n300 = call <extravilib>:"Read.vi"("channel"=w563) -> ("element"=w565:bool)  [unwired: 1 in, 1 out]
                      n301 = Or(x=w566, y=w565) -> (x .or. y?=w564:bool)
                      n302 = Build Array(w558, w551, w550, w549, w548, w547) -> (w546:dbl[])
                      n303 = node-c288() -> ()  [unwired: 1 in, 1 out]
                      n304 = call "LiveDataUpload.vi"("Input Array"=w546, "API String"="API Key") -> ()  [unwired: 10 in]
                    }
                  }
                }
                n305 = node-c288() -> ()  [unwired: 1 in, 1 out]
                n306 = node-c288() -> ()  [unwired: 1 in, 1 out]
              }
              n307 = local read "Hold Time\n[min]"() -> (w245:dbl)
              n308 = Multiply(x=w245, y=60000.0) -> (x*y=w244:dbl)
              n309 = Subtract(x=w244, y=12000.0) -> (x-y=w242:dbl)
              n310 = Divide(x=w242, y="t_read [ms]") -> (x/y=w238:dbl)
              n311 = Round To Nearest(number=w238) -> (nearest integer value=w237:dbl)
              n312 = Subtract(x=w237, y=2.0) -> (x-y=w232:dbl)
              "read_cnt_true" <- w232
              n313 = local read "Hold Time\n[min]"() -> (w234:dbl)
              n314 = local read "t_read [ms]"() -> (w233:dbl)
              n315 = xnode "Formula"("X1"=w234, "X2"=w232, "X3"=w233) -> ("Result"=→"t_diff":dbl)  [unwired: 1 in, 1 out]
              n316 = call <extravilib>:"Read.vi"("channel"=w241) -> ("element"=w248:bool)  [unwired: 1 in, 1 out]
              n317 = Equal?(x=w240, y=0.0) -> (x = y?=w249:bool)
              n318 = Or(x=w249, y=w248) -> (x .or. y?=w247:bool)
              n319 = node-c288(w252) -> ()  [unwired: 1 out]
            }
            n320 = node-c288() -> ()  [unwired: 1 in, 1 out]
          }
        }
      }
      n321 = node-c288() -> ()  [unwired: 1 in, 1 out]
      n322 = node-c288() -> ()  [unwired: 1 in, 1 out]
    }
    n323 = Unbundle("COM Port Settings") -> ("Baud Rate"=w37:T10, "VISA Sesssion In"=w36:refnum<visa-resource-name>)
    n324 = Bundle(cluster=T4 {"Unit ID"="A", "Baud Rate"=enum."19200", "VISA Sesssion In"="COM1"} ("Communication Settings"), "Baud Rate"=w37, "VISA Sesssion In"=w36) -> (w35:T4)  [unwired: 1 in]
    n325 = call "COM Port Initialization.vi"("error in (no error)"=errorcluster {"status"=FALSE, "code"=0, "source"=""}, "Communication Settings"=w35) -> ("error out"=w28:errorcluster, "VISA Session Out"=w27:refnum<visa-resource-name>)  [unwired: 8 in]
    n326 = Cluster To Array(cluster="Device ID's \nto Include:") -> (array=w31:bool[])
    n327 = for {
      N: 6 -> [_]
      tunnel: "ABCDEF" -> [w608]
      tunnel: w31 -> [w601] mode=indexing
      shift-right: [w600] -> _
      shift-left: u16 0 ("length (rest)") -> [w606]
      shift-right: [w605] -> w25
      shift-left: cluster{string, u16}[] [] -> [w604]
      tunnel: w28 -> [w599]
      tunnel: w27 -> [w598]
      tunnel: [w599] -> w18
      tunnel: [w598] -> w26
      i -> [w607]
      # "Generate array of Device ID's, with sequential ID's"
      n328 = Equal?(x=w601, y=TRUE) -> (x = y?=w603:bool)
      n329 = case shown="True" w603 {
        tunnel: w608 -> [_ w619]
        tunnel: w607 -> [_ w618]
        tunnel: w606 -> [w609 w611]
        tunnel: [w610 w614] -> w605
        tunnel: w604 -> [w610 w612]
        tunnel: [w609 w615] -> w600
        frame False {
          # "ID was not included"
        }
        frame True {
          # "ID was included"
          n330 = String Subset(string=w619, offset (0)=w618, length (rest)=1 ("length (rest)")) -> (substring=w616:string)
          n331 = Bundle(w616, "length (rest)"=w611) -> (w613:cluster{string, "length (rest)":u16})  [unwired: 1 in]
          n332 = Increment(x=w611) -> (x+1=w615:u16)
          n333 = Build Array (concatenate)(w612, w613) -> (w614:cluster{string, "length (rest)":u16}[])
        }
      }
    }
    n334 = property on="Active Device" class="Ring (strict)"(error in=w18, "StringsAndValues[]"=w25) -> (error out=w17:errorcluster)  [unwired: 1 in, 1 out]
    n335 = for {
      tunnel: w26 -> [w596]
      tunnel: [w593] -> w22
      tunnel: w17 -> [w597]
      tunnel: [w592] -> w21
      tunnel: w25 -> [w594] mode=indexing
      tunnel: [w595] -> w24 mode=indexing
      tunnel: [w585] -> w23 mode=indexing
      tunnel: [w591] -> w20 mode=indexing
      tunnel: [nan ("Setpoint")] -> w19 mode=indexing
      tunnel: [w584] -> w16 mode=indexing
      # "Get measurement formats, unit ID's and the controller info"
      n336 = Unbundle(w594) -> (w585:string)  [unwired: 1 out]
      n337 = property on="Active Device" class="Ring (strict)" props=["Value"]() -> ()  [unwired: 2 in, 3 out]
      n338 = call "Read Measurement Format.vi"("Unit ID (A)"=w585, "error in"=w597, "VISA Session In"=w596) -> ("error out"=w588:errorcluster, "Data Frame Format"=w595:T11, "VISA Session Out"=w589:refnum<visa-resource-name>)  [unwired: 6 in]
      n339 = call "Read Software Version.vi"("Unit ID (A)"=w585, "error in"=w588, "VISA Session In"=w589) -> ("error out"=w587:errorcluster, "Software Version"=w584:u8, "VISA Session Out"=w586:refnum<visa-resource-name>)  [unwired: 6 in]
      n340 = call "Read Controller Info.vi"("Unit ID (A)"=w585, "error in"=w587, "Software Version"=w584, "VISA Session In"=w586) -> ("error out"=w592:errorcluster, "Controller Info out"=w591:T12, "VISA Session Out"=w593:refnum<visa-resource-name>)  [unwired: 4 in, 1 out]
    }
    n341 = while {
      shift-right: [w656] -> _
      shift-left: 0.0 ("Set Start Time (s)") -> [w659]
      shift-right: [w642] -> w40
      shift-left: w21 -> [w658]
      shift-right: [w623] -> w41
      shift-left: w22 -> [w657]
      tunnel: w23 -> [w621]
      shift-right: [w644] -> _
      shift-left: w24 -> [w651]
      shift-right: [w641] -> _
      shift-left: w20 -> [w639]
      shift-right: [w637] -> _
      shift-left: w19 -> [w636]
      shift-right: [w632] -> _
      shift-left: w16 -> [w632]
      tunnel: w12 -> [w630]
      stop <- w631 stop-if-true
      # "Acquire data for every device ID included at the requested data rate, then display only the selected device's data"
      n342 = call "Elapsed Time"("Set Start Time (s)"=w659) -> ("Get Start Time (s)"=w656:dbl, "Elapsed Time (s)"=w653:dbl)  [unwired: 11 in, 6 out]
      n343 = for {
        shift-right: [w688] -> w650
        shift-left: w658 -> [w691]
        shift-right: [w689] -> w649
        shift-left: w657 -> [w690]
        tunnel: w651 -> [w685] mode=indexing
        tunnel: w621 -> [w684] mode=indexing
        tunnel: [w683] -> w648 mode=indexing
        tunnel: [w682] -> w647 mode=indexing
        tunnel: [w681] -> w646 mode=indexing
        tunnel: [w680] -> w645 mode=indexing
        tunnel: [w679] -> w644 mode=indexing
        # "Acquire data for each device"
        n344 = call "Read Measurements.vi"("error in"=w691, "Data Frame Format In"=w685, "Unit ID (A)"=w684, "VISA Session In"=w690) -> ("error out"=w688:errorcluster, "Data Frame Format Out"=w679:T11, "Data Cluster"=w682:T3, "VISA Session Out"=w689:refnum<visa-resource-name>, "Unknown Dataframe Info"=w687:bool, "Error/Overrange/Unknown String"=w681:string, "Error Present"=w686:bool, "Range Exceeded"=w680:bool)
        n345 = Or(x=w687, y=w686) -> (x .or. y?=w683:bool)
      }
      n346 = local read "Z"() -> (w627:dbl[])
      n347 = Index Array(array=w627, index=1 ("index (row)")) -> (element=w625:dbl)
      "Active Device" <- w625
      n348 = To Long Integer(number=w625) -> (32bit integer=w634:i32)
      n349 = Multiply(x=1000.0 ("y"), y=w653) -> (x*y=→"Elapsed Time [ms]\n(all units)":dbl)
      n350 = Reciprocal(x=w653) -> ()  [unwired: 1 out]
      n351 = Wait (ms)(milliseconds to wait="Minimum time between \nreadings [ms] (all units)") -> ()  [unwired: 1 out]
      n352 = for {
        tunnel: w650 -> [w662]
        tunnel: [w661] -> w643
        tunnel: w649 -> [w663]
        tunnel: [w660] -> w622
        tunnel: w648 -> [w668] mode=indexing
        tunnel: w634 -> [w670]
        tunnel: w647 -> [w667] mode=indexing
        tunnel: w646 -> [w666] mode=indexing
        tunnel: w645 -> [w665] mode=indexing
        i -> [w669]
        # "Iterate over all sets of data, only display the one selected"
        n353 = Equal?(x=w670, y=w669) -> (x = y?=w664:bool)
        n354 = case shown="True" w664 {
          tunnel: w668 -> [_ w678]
          tunnel: w667 -> [_ w673]
          tunnel: w666 -> [_ w677]
          tunnel: w665 -> [_ w676]
          tunnel: w663 -> [w672 w674]
          tunnel: w662 -> [w671 w675]
          tunnel: [w671 w675] -> w661
          tunnel: [w672 w674] -> w660
          frame False {
            # "Do nothing"
          }
          frame True {
            # "Display data"
            "Range Exceeded" <- w676
            "Error Present" <- w678
            "Error Text" <- w677
            "Meas. Data (for active device)" <- w673
          }
        }
      }
      n355 = local read "Z"() -> (w629:dbl[])
      n356 = Index Array(array=w632, index=w634) -> (element=w633:u8)
      n357 = Index Array(array=w636, index=w634) -> (element=w624:dbl)
      n358 = Index Array(array=w629, index=0) -> (element=w620:dbl)
      n359 = Replace Array Subset(array=w636, new element=w620, index=w634) -> (w637:dbl[])
      n360 = Index Array(array=w621, index=w634) -> (element=w635:string)
      n361 = Index Array(array=w639, index=w634) -> (element=w638:T12)
      n362 = call "Write SetPoint_no prev.vi"("Setpoint"=w620, "Previous Setpoint"=w624, "Unit ID (A)"=w635, "error in"=w643, "Software Version"=w633, "Controller Info out"=w638, "VISA Session In"=w622) -> ("error out"=w642:errorcluster, "Controller Info out"=w640:T12, "VISA Session Out"=w623:refnum<visa-resource-name>)  [unwired: 1 in, 1 out]
      n363 = Replace Array Subset(array=w639, new element=w640, index=w634) -> (w641:T13)
      n364 = call <extravilib>:"Read.vi"("channel"=w630) -> ("element"=w631:bool)  [unwired: 1 in, 1 out]
    }
    n365 = while "Hold Setpoints" {
      tunnel: w12 -> [w53]
      stop <- w54 stop-if-true
      n366 = call-poly <vilib>:"Read Delimited Spreadsheet.vi"("file path (dialog if empty)"="Read File", "start of read offset (chars.:0)"=0, "delimiter (\\t)"="," ("delimiter (\\t)")) -> ("all rows"=w49:dbl[][])  [unwired: 7 in, 5 out]
      "all rows" <- w49
      n367 = Array Subset(array=w49, index (row)="Start From:") -> (w47:dbl[][])  [unwired: 3 in]
      "Setpoints" <- w47
      n368 = Array Size(array=w47) -> (size(s)=w56:i32[])
      n369 = Index Array(array=w56, index=0) -> (element=→"len_SP":i32)
      n370 = call <extravilib>:"Read.vi"("channel"=w53) -> ("element"=w54:bool)  [unwired: 1 in, 1 out]
    }
    n371 = VISA Close(VISA resource name=w41, error in (no error)=w40) -> (error out=w42:errorcluster)
    n372 = Initialize Array(0.0 ("element"), 2 ("dimension size")) -> (→"Z":dbl[])
    n373 = call <vilib>:"Simple Error Handler.vi"("error in (no error)"=w42) -> ("error?"=w4:bool)  [unwired: 4 in, 4 out]
    n374 = call "CalibrationAlerts.vi"("Alert Type (0)"=5, "Trigger"=w4) -> ()  [unwired: 10 in]
    n375 = call-poly <vilib>:"Write Delimited Spreadsheet.vi"("file path (dialog if empty)"="Write File", "1D data"=string[] ["Date/Time", "Time [hh:mm:ss]", "Device ID", "P_MFC [psia]", "T_MFC [C]", "Volume Flow [LPM]", "Mass Flow [SLPM]", "SP_MFC [LPM]", "T_SCh [C]", "Iter_#", "V_D [V]", "V_H [V]", "Iter_Duration [ms]", "C_SP_CH4 [ppm]", "C_SP_H2S [ppm]"], "append to file? (new file:F)"=TRUE, "delimiter (\\t)"="," ("delimiter (\\t)")) -> ()  [unwired: 10 in, 2 out]
    n376 = node-c288(w45) -> ()  [unwired: 1 out]
  }
